vi "get wavefront.vi"(8 "error in":errorcluster, 11 "HasoSlopes in":refnum<class "HasoSlopes.lvclass">) -> (0 "error out":errorcluster, 1 "Pupil (new)":refnum<class "Pupil.lvclass">, 2 "Phase":refnum<class "Phase.lvclass">, 3 "HasoData out":refnum<class "HasoData.lvclass">, 5 "ComputePhaseSet.lvclass 2":refnum<class "ComputePhaseSet.lvclass">)   [LabVIEW 2020]
uses:
  WaveKit/Classes/Pupil/Pupil.lvclass
  WaveKit/Classes/Phase/Phase.lvclass
  WaveKit/Classes/HasoSlopes/HasoSlopes.lvclass
  WaveKit/Classes/ComputePhaseSet/ComputePhaseSet.lvclass
  WaveKit/Classes/HasoData/HasoData.lvclass
  WaveKit/Controls/WavefrontReconstructionMode.ctl
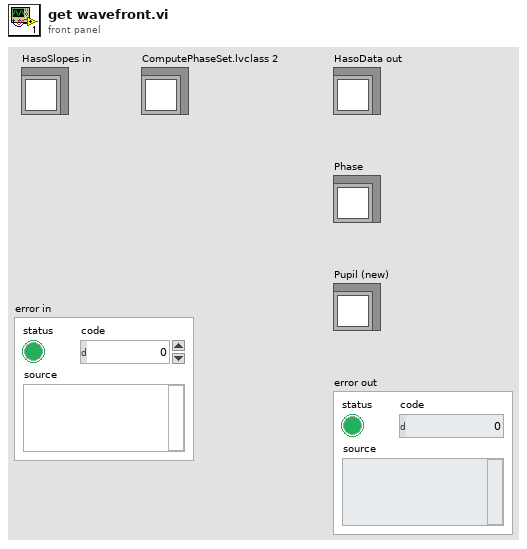
[diagram p1: front panel]
types:
  T1 = typedef "WavefrontReconstructionMode.ctl" = enum16{"None", "Modal_Legendre", "Modal_Zernike", "Zonal", "Modal_Zonal_Zernike", "Modal_Zonal_Legendre"}
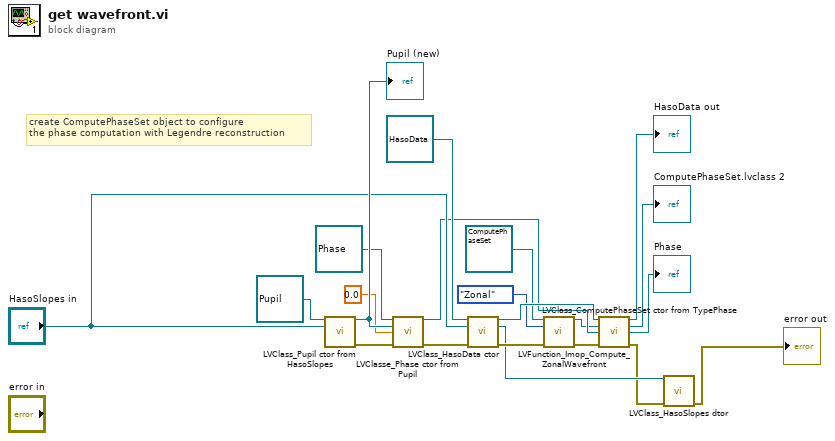
[diagram p0: block diagram]
diagram:
  # "create ComputePhaseSet object to configure\nthe phase computation with Legendre reconstruction"
  n1 = call "LVClass_Pupil ctor from HasoSlopes.vi"("Pupil (const)"=refnum<class "Pupil.lvclass"> refnum ("Pupil in"), "HasoSlopes"="HasoSlopes in") -> ("Pupil (new)"=w21:refnum<class "Pupil.lvclass">, "error out"=w9:errorcluster)  [unwired: 11 in, 1 out]
  "Pupil (new)" <- w21
  n2 = call "LVClasse_Phase ctor from Pupil.vi"("Phase (const)"=refnum<class "Phase.lvclass"> refnum ("Phase in"), "Pupil"=w21, "coef"=sgl 0.0, "error in (no error)"=w9) -> ("Phase (new)"=w11:refnum<class "Phase.lvclass">, "error out"=w15:errorcluster)  [unwired: 9 in, 1 out]
  n3 = call "LVClass_HasoData ctor.vi"("HasoData (const)"=refnum<class "HasoData.lvclass"> refnum ("HasoData in"), "HasoSlopes"="HasoSlopes in", "error in (no error)"=w15) -> ("HasoData (new)"=w18:refnum<class "HasoData.lvclass">, "HasoSlopes (dup)"=w3:refnum<class "HasoSlopes.lvclass">, "error out"=w16:errorcluster)  [unwired: 10 in]
  n4 = call "LVClass_ComputePhaseSet ctor from TypePhase.vi"("ComputePhaseSet (const)"=refnum<class "ComputePhaseSet.lvclass"> refnum ("ComputePhaseSet in"), "TypePhase"=WavefrontReconstructionMode."Zonal", "error in (no error)"=w16) -> ("ComputePhaseSet (new)"=w10:refnum<class "ComputePhaseSet.lvclass">, "error out"=w17:errorcluster)  [unwired: 11 in]
  n5 = call "LVFunction_Imop_Compute_ZonalWavefront.vi"("HasoData.lvclass"=w18, "ComputePhaseSet.lvclass"=w10, "Phase"=w11, "error constant"=w17) -> ("HasoData.lvclass (dup)"=→"HasoData out":refnum<class "HasoData.lvclass">, "ComputePhaseSet.lvclass 2"=→"ComputePhaseSet.lvclass 2":refnum<class "ComputePhaseSet.lvclass">, "Phase"=→"Phase":refnum<class "Phase.lvclass">, "error out"=w2:errorcluster)  [unwired: 8 in]
  n6 = call "LVClass_HasoSlopes dtor.vi"("HasoSlopes in"=w3, "error in (no error)"=w2) -> ("error out"=→"error out":errorcluster)  [unwired: 12 in, 1 out]
